vi "_remove_header_from_maps.vi"(10 "header":string[](array[string]), 11 "httpHeaders in":refnum<class "httpHeaders.lvclass">) -> (3 "httpHeaders out":refnum<class "httpHeaders.lvclass">)   [LabVIEW 2020, in "httpClient.lvlib" / "httpHeaders.lvclass"]
uses:
  httpHeaders.lvclass
  httpHeaders.lvclass/httpHeaders.ctl
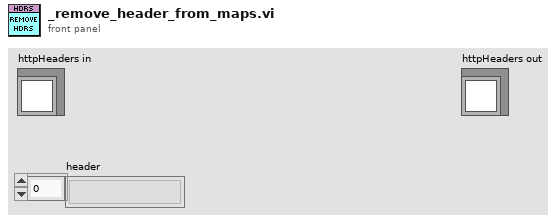
[diagram p1: front panel]
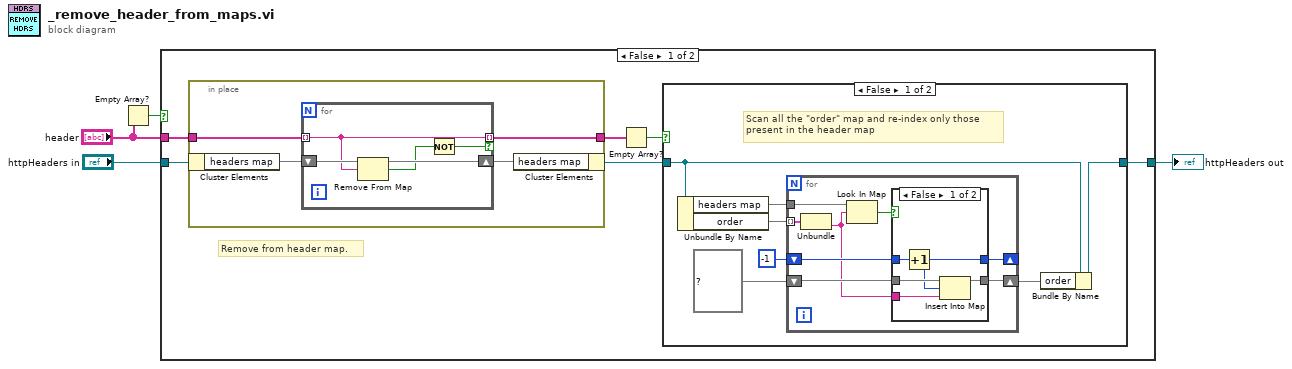
[diagram p0: block diagram]
diagram:
  n1 = Empty Array?(array="header") -> (empty?=w1:bool)
  n2 = case shown="False" w1 {
    tunnel: "httpHeaders in" -> [w10 w43]
    tunnel: [w6 w43] -> w3
    tunnel: "header" -> [w9 _]
    frame False {
      # "Remove from header map."
      n3 = in-place {
        in-place-border: w9 -> [w37]
        in-place-border: [w34] -> w5
        n4 = in-place-cluster #1(w10) -> ("headers map"=w36:map{string, string})
        n5 = for {
          tunnel: w37 -> [w40] mode=indexing
          shift-right: [w41] -> w35
          shift-left: w36 -> [w42]
          tunnel: [w40] -> w34 mode=indexing if=w38
          n6 = Remove From Map(10:w40, 11:w42) -> (2:w39:bool, 3:w41:map{string, string})  [unwired: 1 out]
          n7 = Not(x=w39) -> (.not. x?=w38:bool)
        }
        n8 = in-place-cluster #1("headers map"=w35) -> (w7:refnum<class "httpHeaders.lvclass">)
      }
      n9 = Empty Array?(array=w5) -> (empty?=w8:bool)
      n10 = case shown="False" w8 {
        tunnel: w7 -> [w16 w33]
        tunnel: [w17 w33] -> w6
        frame False {
          # "Scan all the \"order\" map and re-index only those\npresent in the header map"
          n11 = Unbundle By Name(w16) -> ("headers map"=w14:map{string, string}, "order"=w15:map{i32, string})
          n12 = for {
            tunnel: w15 -> [w25] mode=indexing
            tunnel: w14 -> [w24]
            shift-right: [w22] -> w12
            shift-left: map{i32, string} {} ("order") -> [w23]
            shift-right: [w20] -> _
            shift-left: -1 ("index") -> [w21]
            n13 = Unbundle(w25) -> ("key"=w19:string)  [unwired: 1 out]
            n14 = Look In Map(map=w24, key=w19) -> (key not found?=w18:bool)  [unwired: 1 in, 1 out]
            n15 = case shown="False" w18 {
              tunnel: w23 -> [w30 w31]
              tunnel: [w29 w31] -> w22
              tunnel: w21 -> [w28 w32]
              tunnel: [w27 w32] -> w20
              tunnel: w19 -> [w26 _]
              frame False {
                n16 = Increment(x=w28) -> (x+1=w27:i32)
                n17 = Insert Into Map(map in=w30, key=w27, value=w26) -> (map out=w29:map{i32, string})  [unwired: 2 out]
              }
              frame True {
              }
            }
          }
          n18 = Bundle By Name(cluster=w16, "order"=w12) -> (w17:refnum<class "httpHeaders.lvclass">)
        }
        frame True {
          # "No header removed.\nNo need to recalculate\nthe order map"
        }
      }
    }
    frame True {
      # "empty input"
    }
  }
  "httpHeaders out" <- w3
